vi "DFD Convert Structure.vi"(8 "error in (no error)":errorcluster, 10 "target structure":u16(ring)=1 items=["FIR Direct Form"=1, "FIR Direct Form Transposed"=2, "FIR Symmetric"=3, "FIR Antisymmetric"=4, "IIR Direct Form I"=5, "IIR Direct Form I Transposed"=6, "IIR Direct Form II"=7, "IIR Direct Form II Transposed"=8, "IIR Cascaded Second-Order Sections Form I"=9, "IIR Cascaded Second-Order Sections Form I Transposed"=10, "IIR Cascaded Second-Order Sections Form II"=11, "IIR Cascaded Second-Order Sections Form II Transposed"=12, "Lattice Allpass (basic sections)"=13, "Lattice Allpass (one multiplier sections)"=14, "Lattice Allpass (normalized sections)"=15, "Lattice AR (basic sections)"=16, "Lattice AR (one multiplier sections)"=17, "Lattice AR (normalized sections)"=18, "Lattice MA (minimum phase)"=19, "Lattice MA (maximum phase)"=20, "Lattice ARMA (basic sections)"=21, "Lattice ARMA (one multiplier sections)"=22, "Lattice ARMA (normalized sections)"=23], 11 "filter in":T1={"mSRate_Fs"=1.0, "mSRate_Version"="2.0", "mSRate_Comments"="", "mSRate_OrgCoef"={"type"=enum."Undefined", "gain"=1.0, "coef a (k)"=[], "coef b (v)"=[]}, "mSRate_CurCoef"={"type"=enum."Undefined", "gain"=1.0, "coef a (k)"=[], "coef b (v)"=[]}, "mSRate_Quantized?"=FALSE, "mSRate_QCoef"={"type"=enum."Undefined", "gain"=1.0, "coef a (k)"=[], "coef b (v)"=[]}, "mSRate_QSettings"=[], "mSRate_Order"=0, "mSRate_Scaling"={"mSRate_ScaleByPowerOf2?"=FALSE, "mSRate_ScaleType"=enum."No Norm"}} {"mSRate_QSettings"."source" items=["Coef a/k"=0, "Coef b/v"=7, "Input"=1, "Output"=2, "Multiplicand"=3, "Product"=4, "Sum"=5, "Delay"=6, "Gain"=8]}) -> (0 "error out":errorcluster, 3 "filter out":T1={"mSRate_Fs"=1.0, "mSRate_Version"="2.0", "mSRate_Comments"="", "mSRate_OrgCoef"={"type"=enum."Undefined", "gain"=1.0, "coef a (k)"=[], "coef b (v)"=[]}, "mSRate_CurCoef"={"type"=enum."Undefined", "gain"=1.0, "coef a (k)"=[], "coef b (v)"=[]}, "mSRate_Quantized?"=FALSE, "mSRate_QCoef"={"type"=enum."Undefined", "gain"=1.0, "coef a (k)"=[], "coef b (v)"=[]}, "mSRate_QSettings"=[], "mSRate_Order"=0, "mSRate_Scaling"={"mSRate_ScaleByPowerOf2?"=FALSE, "mSRate_ScaleType"=enum."No Norm"}} {"mSRate_QSettings"."source" items=["Coef a/k"=0, "Coef b/v"=7, "Input"=1, "Output"=2, "Multiplicand"=3, "Product"=4, "Sum"=5, "Delay"=6, "Gain"=8]})   [LabVIEW 2017, in "NI_DigFilterLicensed.lvlib"]
doc: "Converts the structure of a filter to a new structure that you specify."
uses:
  <vilib>/addons/Digital Filter Design/NI_DigFilterLicensed.lvlib
  <vilib>/addons/Digital Filter Design/_Objects.llb/DFD Filter Obj.ctl
  <vilib>/addons/Digital Filter Design/_Objects.llb/DFD Filter Coef.ctl
  <vilib>/addons/Digital Filter Design/_Objects.llb/DFD Filter Structure Type Selector.ctl
  <vilib>/addons/Digital Filter Design/_Objects.llb/dfd_Internal Quantization Settings.ctl
  <vilib>/addons/Digital Filter Design/_Objects.llb/dfd_Internal Quantization Srcs.ctl
  <vilib>/addons/Digital Filter Design/_Objects.llb/DFD Coef Norm Type.ctl
  <vilib>/addons/Digital Filter Design/FilterLib.llb/dfd_Set Filter Coef Type (Coef IO).vi
  <vilib>/addons/Digital Filter Design/_Misc.llb/dfd_Error Cluster From Error Code (Scalar).vi
  <vilib>/addons/Digital Filter Design/FilterLib.llb/dfd_Get Filter Coef Type (Filter IO).vi
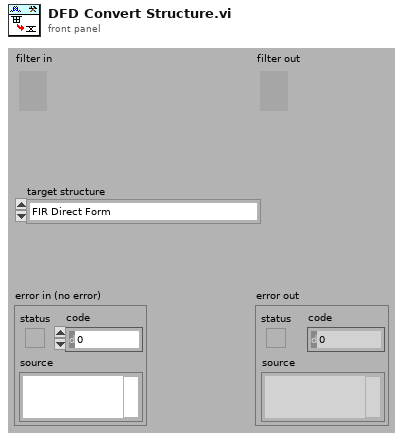
[diagram p1: front panel]
types:
  T1 = typedef "NI_DigFilterLicensed.lvlib/DFD Filter Obj.ctl" = cluster{"mSRate_Fs":dbl, "mSRate_Version":string, "mSRate_Comments":string, "mSRate_OrgCoef":T2, "mSRate_CurCoef":T2, "mSRate_Quantized?":bool, "mSRate_QCoef":T2, "mSRate_QSettings":T4[], "mSRate_Order":i32, "mSRate_Scaling":cluster{"mSRate_ScaleByPowerOf2?":bool, "mSRate_ScaleType":T6}}
  T2 = typedef "NI_DigFilterLicensed.lvlib/DFD Filter Coef.ctl" = cluster{"type":T3, "gain":dbl, "coef a (k)":dbl[], "coef b (v)":dbl[]}
  T3 = typedef "NI_DigFilterLicensed.lvlib/DFD Filter Structure Type Selector.ctl" = enum16{"Undefined", "FIR Direct Form", "FIR Direct Form Transposed", "FIR Symmetric", "FIR Antisymmetric", "IIR Direct Form I", "IIR Direct Form I Transposed", "IIR Direct Form II", "IIR Direct Form II Transposed", "IIR Cascaded Second Order Sections Form I", "IIR Cascaded Second Order Sections Form I Transposed", "IIR Cascaded Second Order Sections Form II", "IIR Cascaded Second Order Sections Form II Transposed", "Lattice Allpass (basic sections)", "Lattice Allpass (one multiplier sections)", "Lattice Allpass (normalized sections)", "Lattice AR (basic sections)", "Lattice AR (one multiplier sections)", "Lattice AR (normalized sections)", "Lattice MA (minimum phase)", "Lattice MA (maximum phase)", "Lattice ARMA (basic sections)", "Lattice ARMA (one multiplier sections)", "Lattice ARMA (normalized sections)"}
  T4 = typedef "NI_DigFilterLicensed.lvlib/dfd_Internal Quantization Settings.ctl" = cluster{"source":T5, "wl":i16, "iwl":i16, "overflow mode":enum16{"Saturation", "Wrap"}, "rounding mode":enum16{"Nearest", "Truncation"}, "signed?":bool}
  T5 = typedef "NI_DigFilterLicensed.lvlib/dfd_Internal Quantization Srcs.ctl" = u16
  T6 = typedef "NI_DigFilterLicensed.lvlib/DFD Coef Norm Type.ctl" = enum16{"No Norm", "Time Domain 1-Norm", "Time Domain 2-Norm", "Time Domain Inf-Norm"}
  T7 = typedef "NI_DigFilterLicensed.lvlib/DFD Filter Structure Id.ctl" = enum16{"Undefined", "FIR", "IIR Direct", "IIR SOS", "IIR Allpass", "IIR AR", "IIR ARMA"}
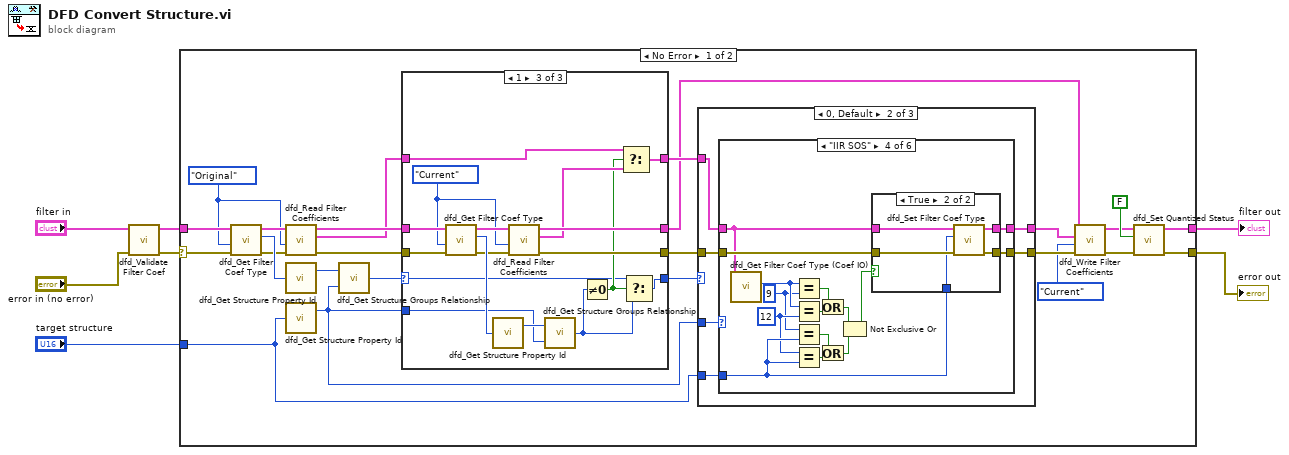
[diagram p0: block diagram]
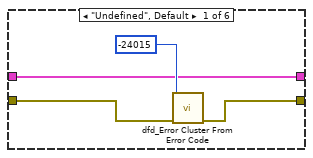
[diagram p3: hidden frame]
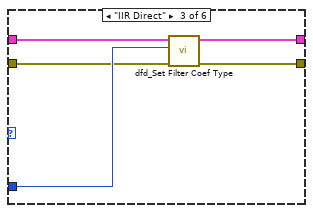
[diagram p5: hidden frame]
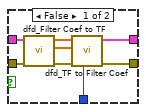
[diagram p6: hidden frame]
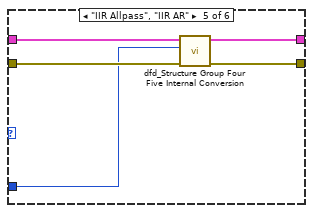
[diagram p7: hidden frame]
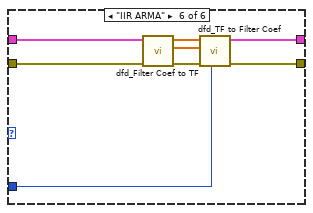
[diagram p8: hidden frame]
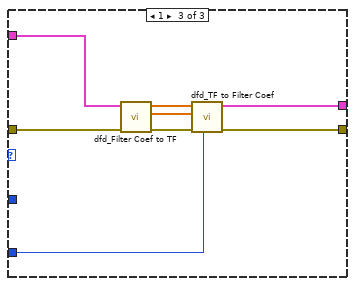
[diagram p9: hidden frame]
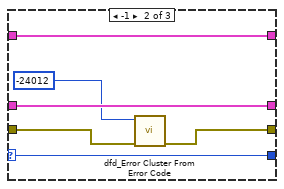
[diagram p11: hidden frame]
diagram:
  n1 = call <vilib>:"dfd_Validate Filter Coef.vi"("error in (no error)"="error in (no error)", "filter in"="filter in") -> ("error out"=w7:errorcluster, "filter out"=w6:T1)  [unwired: 1 in, 7 out]
  n2 = case shown="No Error" w7 {
    selector: w7 -> [w28 w128]
    tunnel: w6 -> [w30 w129]
    tunnel: "target structure" -> [w9 _]
    tunnel: [w21 w129] -> w3
    tunnel: [w22 w128] -> w2
    frame No Error {
      w19 = enum16{"Original", "Current", "Quantized"}."Original" ("coef source")
      n3 = call-poly <vilib>:"dfd_Get Filter Coef Type.vi"("error in (no error)"=w28, "coef source"=w19, "filter in"=w30) -> ("error out"=w25:errorcluster, "type"=w29:T3, "filter out"=w27:T1)  [unwired: 1 in, 5 out]
      n4 = call <vilib>:"dfd_Read Filter Coefficients.vi"("error in (no error)"=w25, "coef source"=w19, "filter in"=w27) -> ("error out"=w23:errorcluster, "filter coef"=w24:T2, "filter out"=w26:T1)  [unwired: 6 out]
      n5 = call <vilib>:"dfd_Get Structure Property Id.vi"("structure type"=w29) -> ("filter structure id"=w31:T7)  [unwired: 1 out]
      n6 = call <vilib>:"dfd_Get Structure Property Id.vi"("structure type"=w9) -> ("filter structure id"=w15:T7)  [unwired: 1 out]
      n7 = call <vilib>:"dfd_Get Structure Groups Relationship.vi"("target group id"=w15, "source group id"=w31) -> ("relationship"=w32:i32)
      n8 = case shown="1" w32 {
        selector: w32 -> [w102 w110 w111]
        tunnel: w26 -> [w104 w109 w127]
        tunnel: w15 -> [_ _ w112]
        tunnel: [w104 w109 w120] -> w8
        tunnel: w24 -> [w101 w108 w118]
        tunnel: w23 -> [w103 w107 w125]
        tunnel: [w103 w106 w119] -> w18
        tunnel: [w101 w108 w115] -> w17
        tunnel: [w102 w110 w114] -> w16
        frame 0, Default {
        }
        frame -1 {
          n9 = call-poly <vilib>:"dfd_Error Cluster From Error Code.vi"("error in (no error)"=w107, "error code (0)"=-24012 ("ERR_INCOMPATIBLE_STRUT")) -> ("error out"=w106:errorcluster)  [unwired: 9 out]
        }
        frame 1 {
          w121 = enum16{"Original", "Current", "Quantized"}."Current" ("coef source")
          n10 = call-poly <vilib>:"dfd_Get Filter Coef Type.vi"("error in (no error)"=w125, "coef source"=w121, "filter in"=w127) -> ("error out"=w122:errorcluster, "type"=w123:T3, "filter out"=w126:T1)  [unwired: 6 out]
          n11 = call <vilib>:"dfd_Get Structure Property Id.vi"("structure type"=w123) -> ("filter structure id"=w124:T7)  [unwired: 1 out]
          n12 = call <vilib>:"dfd_Read Filter Coefficients.vi"("error in (no error)"=w122, "coef source"=w121, "filter in"=w126) -> ("error out"=w119:errorcluster, "filter coef"=w117:T2, "filter out"=w120:T1)  [unwired: 6 out]
          n13 = call <vilib>:"dfd_Get Structure Groups Relationship.vi"("target group id"=w112, "source group id"=w124) -> ("relationship"=w116:i32)
          n14 = Not Equal To 0?(x=w116) -> (x != 0?=w113:bool)
          n15 = Select(t=w118, s=w113, f=w117) -> (s? t:f=w115:T2)
          n16 = Select(t=w111, s=w113, f=w116) -> (s? t:f=w114:i32)
        }
      }
      n17 = case shown="0, Default" w16 {
        tunnel: w9 -> [_ w39 w100]
        tunnel: w18 -> [w34 w38 w99]
        tunnel: [w34 w36 w93] -> w14
        tunnel: w15 -> [_ w40 _]
        tunnel: w17 -> [w33 w37 w95]
        tunnel: [w33 w35 w94] -> w13
        frame -1 {
        }
        frame 0, Default {
          n18 = case shown="\"IIR SOS\"" w40 {
            tunnel: w39 -> [_ _ w51 w57 w83 w88]
            tunnel: w38 -> [w44 w46 w50 w66 w84 w90]
            tunnel: [w41 w45 w47 w64 w82 w85] -> w35
            tunnel: [w43 w46 w49 w65 w81 w87] -> w36
            tunnel: w37 -> [w41 w45 w48 w63 w80 w86]
            frame "Undefined", Default {
              n19 = call-poly <vilib>:"dfd_Error Cluster From Error Code.vi"("error in (no error)"=w44, "error code (0)"=-24015 ("ERR_INVALID_FILTER_OBJ")) -> ("error out"=w43:errorcluster)  [unwired: 9 out]
            }
            frame "FIR" {
            }
            frame "IIR Direct" {
              n20 = call-poly <vilib>:"dfd_Set Filter Coef Type.vi"("error in (no error)"=w50, "type"=w51, "filter coef in"=w48) -> ("error out"=w49:errorcluster, "filter coef out"=w47:T2)  [unwired: 7 out]
            }
            frame "IIR SOS" {
              w56 = u16 12 ("target structure")
              w55 = u16 9 ("target structure")
              n21 = call <vilib>:"dfd_Get Filter Coef Type (Coef IO).vi"("filter coef in"=w63) -> ("type"=w62:T3)  [unwired: 1 in, 9 out]
              n22 = Equal?(x=w62, y=w55) -> (x = y?=w60:bool)
              n23 = Equal?(x=w62, y=w56) -> (x = y?=w61:bool)
              n24 = Equal?(x=w55, y=w57) -> (x = y?=w59:bool)
              n25 = Equal?(x=w56, y=w57) -> (x = y?=w58:bool)
              n26 = Or(x=w60, y=w61) -> (x .or. y?=w54:bool)
              n27 = Or(x=w59, y=w58) -> (x .or. y?=w53:bool)
              n28 = Not Exclusive Or(1:w53, 2:w54) -> (0:w52:bool)
              n29 = case shown="True" w52 {
                tunnel: w66 -> [w68 w79]
                tunnel: [w69 w78] -> w65
                tunnel: w63 -> [w71 w77]
                tunnel: [w70 w76] -> w64
                tunnel: w57 -> [w67 w75]
                frame False {
                  n30 = call <vilib>:"dfd_Filter Coef to TF.vi"("error out"=w68, "filter coef"=w71) -> ("error"=w73:errorcluster, "denominator"=w74:dbl[], "numerator"=w72:dbl[])  [unwired: 7 out]
                  n31 = call <vilib>:"dfd_TF to Filter Coef.vi"("type"=w67, "error in (no error)"=w73, "denominator"=w74, "numerator"=w72) -> ("error out"=w69:errorcluster, "filter coef"=w70:T2)  [unwired: 6 out]
                }
                frame True {
                  n32 = call-poly <vilib>:"dfd_Set Filter Coef Type.vi"("error in (no error)"=w79, "type"=w75, "filter coef in"=w77) -> ("error out"=w78:errorcluster, "filter coef out"=w76:T2)  [unwired: 7 out]
                }
              }
            }
            frame "IIR Allpass", "IIR AR" {
              n33 = call <vilib>:"dfd_Structure Group Four Five Internal Conversion.vi"("error in (no error)"=w84, "target structure"=w83, "filter coef in"=w80) -> ("error out"=w81:errorcluster, "filter coef out"=w82:T2)  [unwired: 7 out]
            }
            frame "IIR ARMA" {
              n34 = call <vilib>:"dfd_Filter Coef to TF.vi"("error out"=w90, "filter coef"=w86) -> ("error"=w91:errorcluster, "denominator"=w92:dbl[], "numerator"=w89:dbl[])  [unwired: 7 out]
              n35 = call <vilib>:"dfd_TF to Filter Coef.vi"("type"=w88, "error in (no error)"=w91, "denominator"=w92, "numerator"=w89) -> ("error out"=w87:errorcluster, "filter coef"=w85:T2)  [unwired: 6 out]
            }
          }
        }
        frame 1 {
          n36 = call <vilib>:"dfd_Filter Coef to TF.vi"("error out"=w99, "filter coef"=w95) -> ("error"=w96:errorcluster, "denominator"=w97:dbl[], "numerator"=w98:dbl[])  [unwired: 7 out]
          n37 = call <vilib>:"dfd_TF to Filter Coef.vi"("type"=w100, "error in (no error)"=w96, "denominator"=w97, "numerator"=w98) -> ("error out"=w93:errorcluster, "filter coef"=w94:T2)  [unwired: 6 out]
        }
      }
      n38 = call <vilib>:"dfd_Write Filter Coefficients.vi"("error in (no error)"=w14, "coef source"=enum16{"Original", "Current", "Quantized"}."Current", "filter coef"=w13, "filter in"=w8) -> ("error out"=w10:errorcluster, "filter out"=w11:T1)  [unwired: 6 out]
      n39 = call <vilib>:"dfd_Set Quantized Status.vi"("error in (no error)"=w10, "quantized?"=FALSE, "filter in"=w11) -> ("error out"=w22:errorcluster, "filter out"=w21:T1)  [unwired: 7 out]
    }
    frame Error {
    }
  }
  "filter out" <- w3
  "error out" <- w2
